vi "Calculate Setpoint.vi"(8 "error in (no error)":errorcluster, 10 "time (sec)":dbl, 11 "IA Test Parameters in":refnum<class "IA Test Parameters.lvclass">) -> (0 "error out":errorcluster, 2 "setpoint":dbl, 3 "IA Test Parameters out":refnum<class "IA Test Parameters.lvclass">, 5 "testing?":bool)   [LabVIEW 2020, in "IA Test Parameters.lvclass"]
uses:
  IA Test Parameters.lvclass
  IA Test Parameters.lvclass/IA Test Parameters.ctl
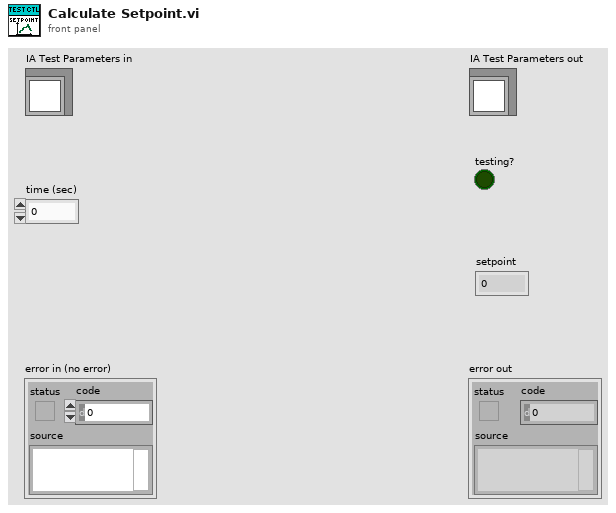
[diagram p1: front panel]
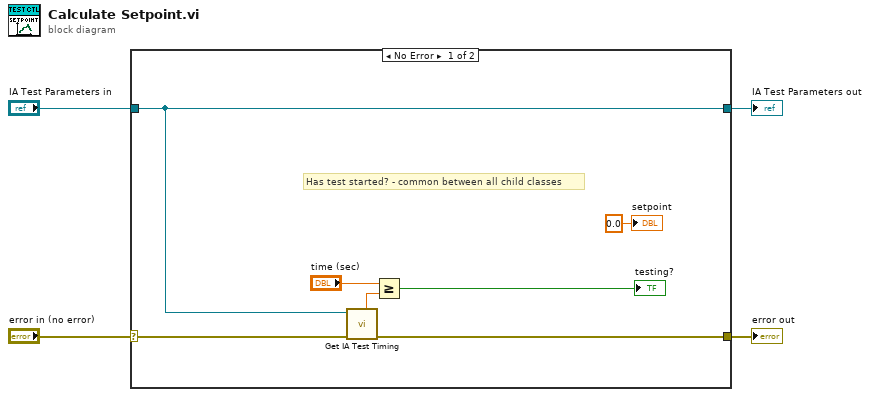
[diagram p0: block diagram]
diagram:
  n1 = case shown="No Error" "error in (no error)" {
    selector: "error in (no error)" -> [w11 w13]
    tunnel: [w10 w13] -> w3
    tunnel: [w9 w12] -> w1
    tunnel: "IA Test Parameters in" -> [w9 w12]
    frame No Error {
      # "Has test started? - common between all child classes"
      n2 = call "Get IA Test Timing.vi"("error in (no error)"=w11, "IA Test Parameters in"=w9) -> ("error out"=w10:errorcluster, "time delay (sec)"=w8:dbl)  [unwired: 4 in, 4 out]
      n3 = Greater Or Equal?(x="time (sec)", y=w8) -> (x >= y?=→"testing?":bool)
      "setpoint" <- 0.0 ("setpoint")
    }
    frame Error {
    }
  }
  "error out" <- w3
  "IA Test Parameters out" <- w1
